vi "VCS Read CAN Frame.vi"(6 "error in (no error)":errorcluster, 7 "timeout":u32, 8 "CAN info":cluster{"cobId":u16, "length":u16}, 9 "keyHandle in":u32) -> (0 "error out":errorcluster, 1 "data":u8[](array[numeric]), 3 "keyHandle out":u32)   [LabVIEW 2017, in "maxonEPOS.lvlib"]
doc: "Function <B>VCS_ReadCANFrame</B> reads a general CAN Frame from the CAN bus."
uses:
  Examples/maxonEPOS.lvlib
  SSI_Tool/InstrumentsInterfaces/Motordriver/maxon EPOS/Resources/EposCmd.dll
  SSI_Tool/InstrumentsInterfaces/Motordriver/maxon EPOS/Resources/EposCmd64.dll
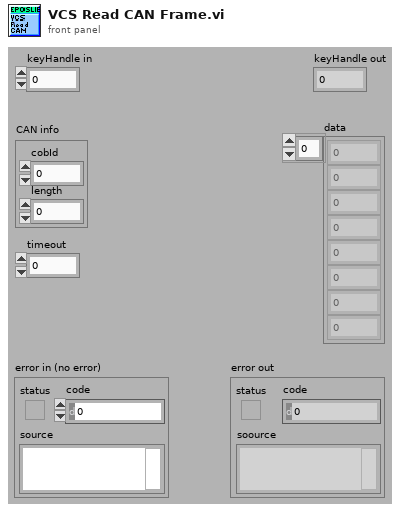
[diagram p1: front panel]
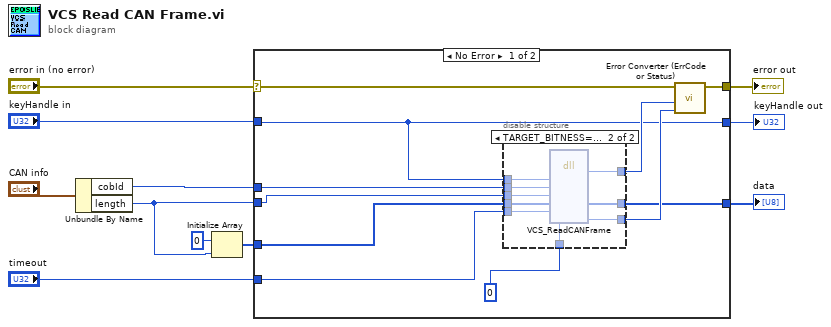
[diagram p0: block diagram]
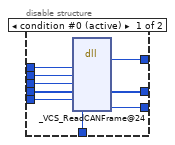
[diagram p2: hidden frame]
diagram:
  n1 = Unbundle By Name("CAN info") -> ("cobId"=w3:u16, "length"=w2:u16)
  n2 = Initialize Array(u8 0, w2) -> (w7:u8[])
  n3 = case shown="No Error" "error in (no error)" {
    selector: "error in (no error)" -> [w21 w43]
    tunnel: [w22 w43] -> w11
    tunnel: [w17 w42] -> w9
    tunnel: w7 -> [w16 w42]
    tunnel: "keyHandle in" -> [w15 w41]
    tunnel: [w15 w41] -> w5
    tunnel: w3 -> [w14 _]
    tunnel: w2 -> [w13 _]
    tunnel: "timeout" -> [w12 _]
    frame No Error {
      n4 = disable-structure shown="TARGET_BITNESS==64" {
        disable-tunnel: u32 0 ("pErrorCode") -> [w31 w40]
        disable-tunnel: [w30 w39] -> w19
        disable-tunnel: [w29 w38] -> w18
        disable-tunnel: [w28 w37] -> w17
        disable-tunnel: w16 -> [w27 w36]
        disable-tunnel: w15 -> [w26 w35]
        disable-tunnel: w14 -> [w25 w34]
        disable-tunnel: w13 -> [w24 w33]
        disable-tunnel: w12 -> [w23 w32]
        frame condition #0 (active) {
          n5 = dll-call lib="C:/workspace/project/scancon/sw/SSI_Tool/InstrumentsInterfaces/Motordriver/maxon EPOS/Resources/EposCmd.*" fn="_VCS_ReadCANFrame@24"("KeyHandle"=w26, "CobID"=w25, "Length"=w24, "pData"=w27, "Timeout"=w23, "pErrorCode"=w31) -> ("Rückgabetyp"=w29:i32, "pData"=w28:u8[], "pErrorCode"=w30:u32)  [unwired: 7 in, 2 out]
        }
        frame condition #1 {
          n6 = dll-call lib="C:/setup/Resources/EposCmd64.*" fn="VCS_ReadCANFrame" ("EposCmd.dll:_VCS_ReadCANFrame@24")("KeyHandle"=w35, "CobID"=w34, "Length"=w33, "pData"=w36, "Timeout"=w32, "pErrorCode"=w40) -> ("Rückgabetyp"=w38:i32, "pData"=w37:u8[], "pErrorCode"=w39:u32)  [unwired: 7 in, 2 out]
        }
      }
      n7 = call "Error Converter (ErrCode or Status).vi"("error code"=w19, "return type"=w18, "error in (no error)"=w21) -> ("error out"=w22:errorcluster)  [unwired: 7 in]
    }
    frame Error {
    }
  }
  "error out" <- w11
  "data" <- w9
  "keyHandle out" <- w5
